vi "Prepend BOM.vi"(8 "error in":errorcluster, 10 "Input Encoding (UTF-16LE)":T1=enum."UTF-16LE", 11 "String":string) -> (0 "error out":errorcluster, 3 "String with BOM":string)   [LabVIEW 2020, in "G-Unicode.lvlib"]
doc: "Prepends the text in <b>String</b> with the Byte Order Mark (BOM) corresponding to the encoding in <b>Input Encoding</b>. If String already contains a BOM, or Input Encoding isn't unicode (UTF-8/UTF-16), <b>String with BOM</b> will be unchanged.\n\nIf the input string encoding isn't known, Input Encoding can be set to Unknown to try and automatically detect the encoding method. Note that automatic encoding detection isn't 100% accurate, and it is recommended to set the encoding explicitly if it is known."
uses:
  G-Unicode.lvlib
  Controls/String Encoding.ctl
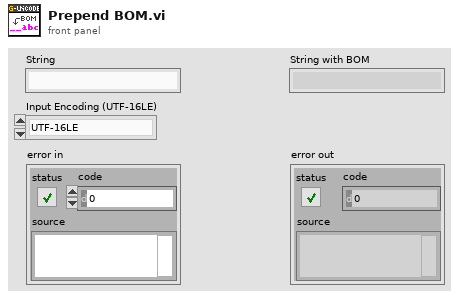
[diagram p1: front panel]
types:
  T1 = typedef "G-Unicode.lvlib/String Encoding.ctl" = enum16{"ANSI", "UTF-8", "UTF-16LE", "UTF-16BE", "Unknown"}
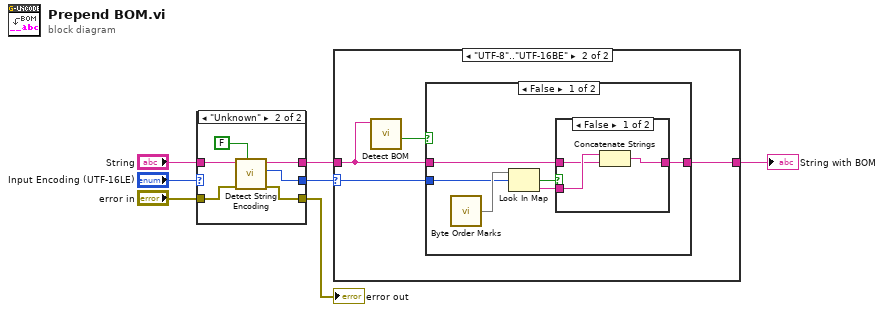
[diagram p0: block diagram]
diagram:
  n1 = case shown="\"Unknown\"" "Input Encoding (UTF-16LE)" {
    selector: "Input Encoding (UTF-16LE)" -> [w8 _]
    tunnel: "String" -> [w10 w16]
    tunnel: [w8 w15] -> w4
    tunnel: [w10 w14] -> w3
    tunnel: "error in" -> [w9 w12]
    tunnel: [w9 w11] -> w1
    frame Default {
    }
    frame "Unknown" {
      n2 = call "Detect String Encoding.vi"("Strip BOM (T)"=FALSE ("Remove BOM (T)"), "error in"=w12, "String"=w16) -> ("error out"=w11:errorcluster, "Encoding"=w15:T1, "String out"=w14:string)  [unwired: 6 in]
    }
  }
  "error out" <- w1
  n3 = case shown="\"UTF-8\"..\"UTF-16BE\"" w4 {
    selector: w4 -> [_ w20]
    tunnel: w3 -> [w17 w21]
    tunnel: [w17 w19] -> w7
    frame Default {
    }
    frame "UTF-8".."UTF-16BE" {
      n4 = call "Detect BOM.vi"("String"=w21) -> ("BOM Found"=w18:bool)  [unwired: 9 in, 1 out]
      n5 = case shown="False" w18 {
        tunnel: w21 -> [w23 w32]
        tunnel: w20 -> [w26 _]
        tunnel: [w22 w32] -> w19
        frame False {
          n6 = call "Byte Order Marks.vi"() -> ("BOMs"=w27:map{T1, string})
          n7 = Look In Map(map=w27, key=w26) -> (key not found?=w25:bool, value=w24:string)  [unwired: 1 in]
          n8 = case shown="False" w25 {
            tunnel: w24 -> [w30 _]
            tunnel: w23 -> [w29 w31]
            tunnel: [w28 w31] -> w22
            frame False {
              n9 = Concatenate Strings(w30, w29) -> (w28:string)
            }
            frame True {
            }
          }
        }
        frame True {
          # "Already has a BOM"
        }
      }
    }
  }
  "String with BOM" <- w7
